vi "Run Test - Axis Selection (SubVI).vi"() -> ()   [LabVIEW 2019]
panel:
  in  "2nd Y-Axis":u16(ring)
  in  "Enable 2nd Y-Axis":bool
  in  "Cancel":bool
  in  "Set":bool
  in  "Y-Axis":u16(ring)
  in  "X-Axis":u16(ring)
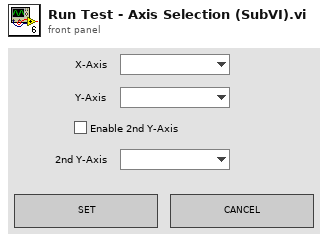
[diagram p1: front panel]
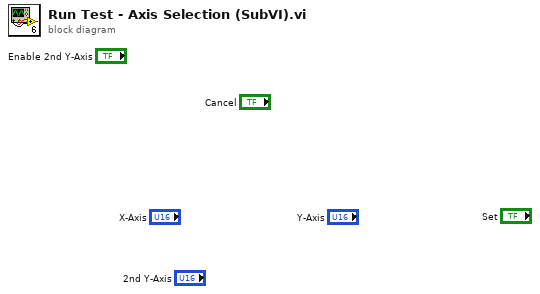
[diagram p0: block diagram]
diagram:
